vi "Initialize UniCyRO Sim.vi"(8 "error in (no error)":errorcluster, 10 "robot ID":string, 11 "UniCyRO_Host_Sim in":refnum<class "UniCyRO_Host_Sim.lvclass">) -> (0 "error out":errorcluster, 3 "UniCyRO_Host_Sim out":refnum<class "UniCyRO_Host_Sim.lvclass">)   [LabVIEW 2012, in "UniCyRO.lvlib" / "UniCyRO_Host_Sim.lvclass"]
uses:
  UniCyRO_Host_Sim.lvclass
  <vilib>/robotics/Simulator/Engine/ctl/DeviceID.ctl
  <vilib>/robotics/Utilities/NI_Robotics Utilities.lvlib
  <vilib>/robotics/Simulator/NI_Robotics_Simulator.lvlib
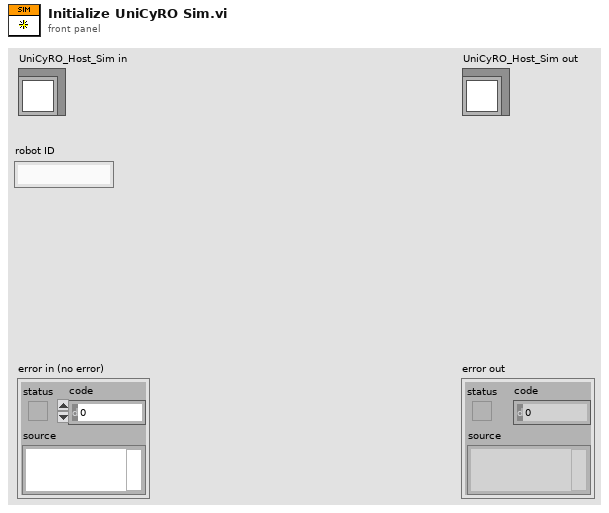
[diagram p1: front panel]
types:
  T1 = typedef "NI_Robotics_Simulator.lvlib/DeviceID.ctl" = cluster{"robot ID":string, "sensor/actuator ID":string}
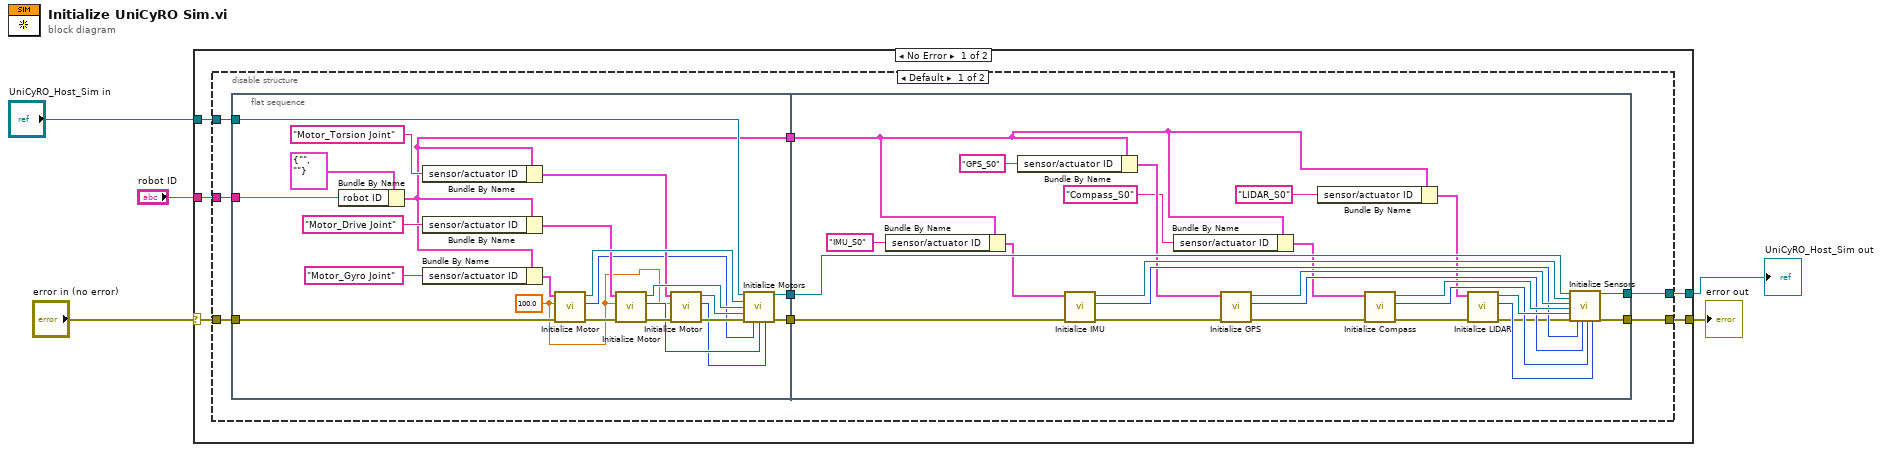
[diagram p0: block diagram]
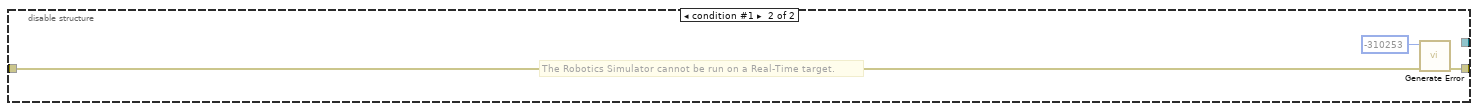
[diagram p2: hidden frame]
diagram:
  n1 = case shown="No Error" "error in (no error)" {
    selector: "error in (no error)" -> [w10 w71]
    tunnel: [w9 w71] -> w4
    tunnel: [w6 w70] -> w2
    tunnel: "UniCyRO_Host_Sim in" -> [w7 w70]
    tunnel: "robot ID" -> [w8 _]
    frame No Error {
      n2 = disable-structure shown="Default" {
        disable-tunnel: w10 -> [w16 w68]
        disable-tunnel: [w12 w67] -> w9
        disable-tunnel: w8 -> [w17 _]
        disable-tunnel: w7 -> [w18 _]
        disable-tunnel: [w13 _] -> w6
        frame condition #0 (active) {
          n3 = flat-sequence {
            tunnel: w18 -> [w39]
            tunnel: w17 -> [w21]
            tunnel: w16 -> [w35]
            tunnel: [w38] -> w15
            tunnel: [w36] -> w14
            tunnel: [w23] -> w11
            tunnel: w15 -> [w65]
            tunnel: w14 -> [w52]
            tunnel: [w66] -> w13
            tunnel: [w51] -> w12
            tunnel: w11 -> [w50]
            frame #0 {
              w19 = sgl 100.0 ("Axis:FMax")
              n4 = Bundle By Name(cluster=T1 {"robot ID"="", "sensor/actuator ID"=""} ("Device ID"), "robot ID"=w21) -> (w23:T1)
              n5 = Bundle By Name(cluster=w23, "sensor/actuator ID"="Motor_Torsion Joint") -> (w27:T1)
              n6 = Bundle By Name(cluster=w23, "sensor/actuator ID"="Motor_Drive Joint") -> (w28:T1)
              n7 = Bundle By Name(cluster=w23, "sensor/actuator ID"="Motor_Gyro Joint") -> (w20:T1)
              n8 = call "Initialize Motor.vi"("error in (no error)"=w35, "Axis:FMax"=w19, "Device ID"=w20) -> ("error out"=w34:errorcluster, "Motor Error"=w26:i32, "DC Motor Controller out"=w29:refnum<class "DC Motor Controller.lvclass">)  [unwired: 6 in]
              n9 = call "Initialize Motor.vi"("error in (no error)"=w34, "Axis:FMax"=w19, "Device ID"=w28) -> ("error out"=w33:errorcluster, "Motor Error"=w25:i32, "DC Motor Controller out"=w30:refnum<class "DC Motor Controller.lvclass">)  [unwired: 6 in]
              n10 = call "Initialize Motor.vi"("error in (no error)"=w33, "Axis:FMax"=w19, "Device ID"=w27) -> ("error out"=w32:errorcluster, "Motor Error"=w24:i32, "DC Motor Controller out"=w31:refnum<class "DC Motor Controller.lvclass">)  [unwired: 6 in]
              n11 = call "Initialize Motors.vi"("UniCyRO_Host_Sim in"=w39, "Gyro Motor"=w29, "Drive Motor"=w30, "Torsion Motor"=w31, "error in (no error)"=w32, "Gyro Motor Error"=w26, "Drive Motor Error"=w25, "Torsion Motor Error"=w24) -> ("UniCyRO_Host_Sim out"=w38:refnum<class "UniCyRO_Host_Sim.lvclass">, "error out"=w36:errorcluster)  [unwired: 6 in]
            }
            frame #1 {
              n12 = Bundle By Name(cluster=w50, "sensor/actuator ID"="IMU_S0") -> (w49:T1)
              n13 = Bundle By Name(cluster=w50, "sensor/actuator ID"="GPS_S0") -> (w48:T1)
              n14 = call "Initialize IMU.vi"("error in (no error)"=w52, "Device ID"=w49) -> ("error out"=w53:errorcluster, "Sensor Error"=w57:i32, "Sparkfun Atomic IMU out"=w61:refnum<class "Sparkfun Atomic IMU.lvclass">)  [unwired: 7 in]
              n15 = Bundle By Name(cluster=w50, "sensor/actuator ID"="Compass_S0") -> (w47:T1)
              n16 = call "Initialize GPS.vi"("error in (no error)"=w53, "Device ID"=w48) -> ("error out"=w54:errorcluster, "Sensor Error"=w58:i32, "Garmin GPS Series out"=w62:refnum<class "Garmin GPS Series.lvclass">)  [unwired: 7 in]
              n17 = Bundle By Name(cluster=w50, "sensor/actuator ID"="LIDAR_S0") -> (w46:T1)
              n18 = call "Initialize Compass.vi"("error in (no error)"=w54, "Device ID"=w47) -> ("error out"=w55:errorcluster, "Sensor Error"=w59:i32, "Honeywell Compass HMC6343"=w63:refnum<class "Honeywell Compass HMC6343.lvclass">)  [unwired: 7 in]
              n19 = call "Initialize LIDAR.vi"("error in (no error)"=w55, "Device ID"=w46) -> ("error out"=w56:errorcluster, "Sensor Error"=w60:i32, "Hokuyo URG Series out"=w64:refnum<class "Hokuyo URG Series.lvclass">)  [unwired: 7 in]
              n20 = call "Initialize Sensors.vi"("UniCyRO_Host_Sim in"=w65, "Sparkfun Atomic IMU out"=w61, "Garmin GPS Series out"=w62, "Honeywell Compass HMC6343"=w63, "Hokuyo URG Series out"=w64, "error in (no error)"=w56, "IMU Error"=w57, "GPS Error"=w58, "Compass Error"=w59, "LIDAR Error"=w60) -> ("UniCyRO_Host_Sim out"=w66:refnum<class "UniCyRO_Host_Sim.lvclass">, "error out"=w51:errorcluster)  [unwired: 8 in]
            }
          }
        }
        frame condition #1 {
          # "The Robotics Simulator cannot be run on a Real-Time target."
          n21 = call <vilib>:"Generate Error.vi"("error in (no error)"=w68, "code"=-310253) -> ("error out"=w67:errorcluster)  [unwired: 9 in]
        }
      }
    }
    frame Error {
    }
  }
  "error out" <- w4
  "UniCyRO_Host_Sim out" <- w2
